vi "SlideOver.vi"(2 "Location":cluster{"X":sgl, "Y":sgl, "Z":sgl}, 3 "Scene.Object IN":refnum<vi>) -> (1 "Scene.Object Out":refnum<vi>)   [LabVIEW 2010]
uses:
  <vilib>/Utility/miscctls.llb/LV3DPointTypeDef.ctl
  LVPresent_Globals.vi
  <vilib>/picture/3D Picture Control/NI_3D Picture Control.lvlib
panel:
  out "Starting Point":T1
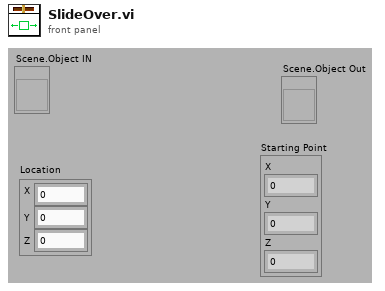
[diagram p1: front panel]
types:
  T1 = typedef "LV3DPointTypeDef.ctl" = cluster{"X":sgl, "Y":sgl, "Z":sgl}
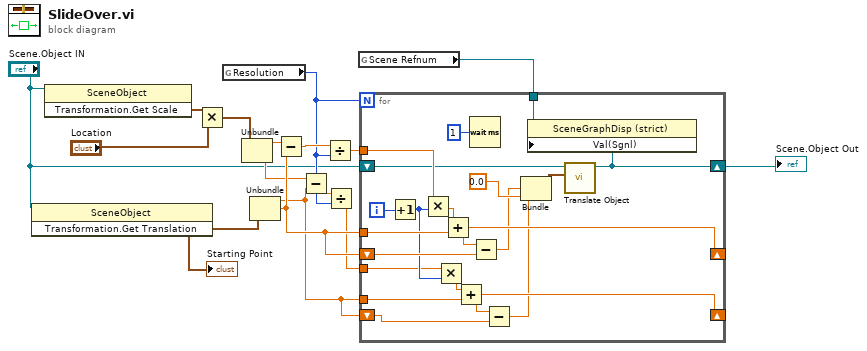
[diagram p0: block diagram]
diagram:
  n1 = invoke class="SceneObject" method="Transformation.Get Translation"(reference="Scene.Object IN") -> ("Transformation.GetTranslation"=w15:T1)  [unwired: 2 in, 2 out]
  "Starting Point" <- w15
  n2 = invoke class="SceneObject" method="Transformation.Get Scale"(reference="Scene.Object IN") -> ("Transformation.Get Scale"=w3:T1)  [unwired: 2 in, 2 out]
  n3 = Multiply(x=w3, y="Location") -> (x*y=w1:T1)
  n4 = global read "LVPresent_Globals.vi" "Resolution"() -> (w7:i32)
  n5 = Unbundle(w1) -> ("X"=w5:sgl, "Y"=w6:sgl)  [unwired: 1 out]
  n6 = Unbundle(w15) -> ("X"=w9:sgl, "Y"=w12:sgl)  [unwired: 1 out]
  n7 = Subtract(x=w5, y=w12) -> (x-y=w13:sgl)
  n8 = Subtract(x=w6, y=w9) -> (x-y=w11:sgl)
  n9 = Divide(x=w13, y=w7) -> (x/y=w14:sgl)
  n10 = Divide(x=w11, y=w7) -> (x/y=w10:sgl)
  n11 = global read "LVPresent_Globals.vi" "Scene Refnum"() -> (w8:refnum<vi>)
  n12 = for {
    N: w7 -> [_]
    shift-right: [w17] -> w16
    shift-left: "Scene.Object IN" -> [w29]
    tunnel: w14 -> [w34]
    tunnel: w12 -> [w25]
    tunnel: w8 -> [w33]
    shift-right: [w27] -> _
    shift-left: w12 -> [w28]
    tunnel: w10 -> [w22]
    tunnel: w9 -> [w21]
    shift-right: [w20] -> _
    shift-left: w9 -> [w19]
    i -> [w36]
    n13 = Increment(x=w36) -> (x+1=w23:i32)
    n14 = Multiply(x=w34, y=w23) -> (x*y=w35:sgl)
    n15 = Multiply(x=w22, y=w23) -> (x*y=w24:sgl)
    n16 = Add(x=w35, y=w25) -> (x+y=w27:sgl)
    n17 = Add(x=w24, y=w21) -> (x+y=w20:sgl)
    n18 = Wait (ms)(milliseconds to wait=u32 1) -> ()  [unwired: 1 out]
    n19 = Subtract(x=w27, y=w28) -> (x-y=w26:sgl)
    n20 = Subtract(x=w20, y=w19) -> (x-y=w18:sgl)
    n21 = Bundle(w18, w26, "Final Zoom"=sgl 0.0) -> (w31:cluster{sgl, sgl, "Final Zoom":sgl})  [unwired: 1 in]
    n22 = call <vilib>:"Translate Object.vi"("Translation"=w31, "Scene.Object In"=w29) -> ("Scene.Object Out"=w17:refnum<vi>)  [unwired: 8 in, 1 out]
    n23 = property class="SceneGraphDisp (strict)"(reference=w33, "Val(Sgnl)"=w17) -> ()  [unwired: 1 in, 2 out]
  }
  "Scene.Object Out" <- w16
